vi "test.vi"() -> ()   [LabVIEW 2014]
panel:
  out "new picture":picture
  in  "py":i64=128
  in  "px":i64=8
  out "index of element":i32
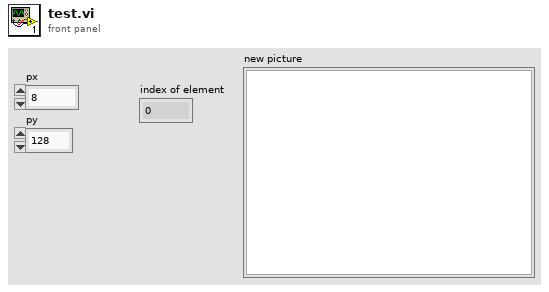
[diagram p1: front panel]
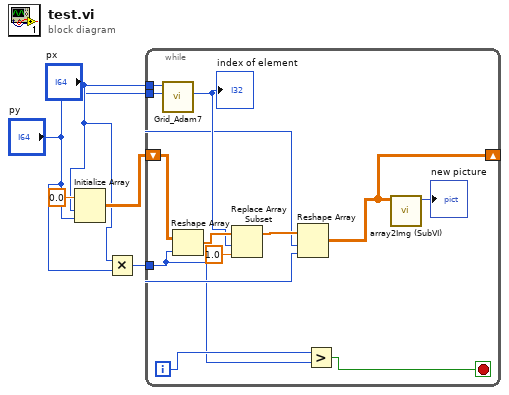
[diagram p0: block diagram]
diagram:
  n1 = Initialize Array(0.0 ("element"), "px", "py") -> (w4:dbl[][])
  n2 = Multiply(x="px", y="py") -> (x*y=w3:i64)
  n3 = while {
    tunnel: w3 -> [w7]
    tunnel: "px" -> [w12]
    tunnel: "py" -> [w11]
    shift-right: [w9] -> _
    shift-left: w4 -> [w17]
    i -> [w8]
    stop <- w6 stop-if-true
    n4 = call "Grid_Adam7.vi"("py 2"=w11, "px 2"=w12) -> ("index of element"=w14:i32)  [unwired: 8 in, 1 out]
    "index of element" <- w14
    n5 = Reshape Array(w17, w7) -> (w15:dbl[])
    n6 = Replace Array Subset(array=w15, new element=1.0 ("new element/subarray"), index=w14) -> (w16:dbl[])
    n7 = Reshape Array(w16, w12, w11) -> (w9:dbl[][])
    n8 = Greater?(x=w8, y=w7) -> (0:w6:bool)
    n9 = call "array2Img (SubVI).vi"("Rxy"=w9) -> ("new picture"=→"new picture":picture)  [unwired: 10 in]
  }
